vi "FTPGlobals.vi"() -> ()   [LabVIEW 2012]
panel:
  out "StatusBar":refnum<vi>
  out "Prefix":string="ME184"
  in  "LocalServerMode?":bool
  out "Username":string
  in  "Default Prefs":string="<?xml version=\"1.0\"?>\n<preferences>\n  <productname>ME-184 RoboBooks</productname>\n  <!-- <productname>LEGO Labs</productname> -->\n  <server>\n    <localhost>localhost</localhost>\n\t<localport>6263</localport>\n\t<remotehost>localhost</remotehost>\n\t<remoteport>57139</remoteport>\n\t<timeout>1000</timeout>\n\t<FIFOSize>100</FIFOSize>\n\t<username></username>\n\t<prefix></prefix>\n  </server>\n  <shelves>\n    <type>ME-184</type>\n    <!-- <type>LEGO Labs</type> -->\n    <resize>false</resize>\n\t<move>false</move>\n  </shelves>\n  <interact>\n    <textbox>HTML</textbox>\n  </interact>\n  <customize>\n\t<grid><size>20</size></grid>\n  </customize>\n</preferences>"
  in  "FIFO Size":i16=100
  out "win ID":i32
  out "OS Name":string
  in  "Paths":T1={"Root"=path "/Kimberly/Applications/ROBOLAB 2.9/vi.lib/RoboBookEngine/RootFolder", "Shelves"=path "/Kimberly/Users/crogers/Documents/ROBOLAB Data/RoboBooks/Shelves", "Cmds"=path "/Kimberly/Applications/ROBOLAB 2.9/vi.lib/RoboBookEngine/HTTPServer/ServerCommands", "Plugins"=path "/Kimberly/Applications/ROBOLAB 2.9/vi.lib/RoboBookEngine/HTTPServer/ServerCommands"}
  in  "ServerInfo":T2={"HostName or IP"="127.0.0.1", "ListeningPort"=6263, "remote address"="localhost", "remote port"=57139}
  in  "TCP Timeout":i32=500
  in  "Last Write":timestamp=timestamp(3310892800.601883 s since 1904-01-01) format="%<%.3X>T"
  in  "Last Read":timestamp=timestamp(3310892800.441162 s since 1904-01-01) format="%<%.3X>T"
  in  "Last Timeout":timestamp=timestamp(3310892818.7440033 s since 1904-01-01) format="%<%.3X>T"
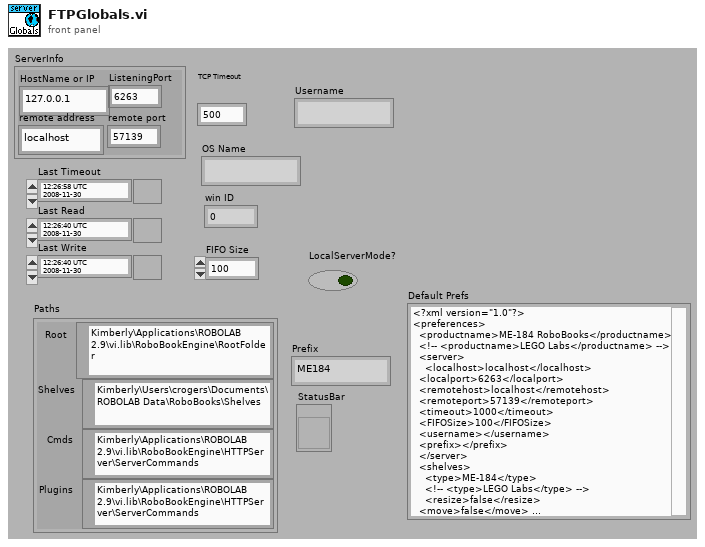
[diagram p1: front panel]
types:
  T1 = cluster{"Root":path, "Shelves":path, "Cmds":path, "Plugins":path}
  T2 = cluster{"HostName or IP":string, "ListeningPort":u16, "remote address":string, "remote port":u16}
diagram:
